vi "Init Waveform.vi"(8 "error in (no error)":errorcluster, 11 "DAQmx Synthesizer in":refnum<class "DAQmx Synthesizer.lvclass">) -> (0 "error out":errorcluster, 3 "DAQmx Synthesizer out":refnum<class "DAQmx Synthesizer.lvclass">)   [LabVIEW 2021, in "DAQmx Synthesizer.lvclass"]
uses:
  DAQmx Synthesizer.lvclass
  DAQmx Synthesizer.lvclass/DAQmx Synthesizer.ctl
  <vilib>/Waveform/WDTOps.llb/WDT Waveform Duration DBL.vi
  <vilib>/Waveform/WDTOps.llb/WDT Get Waveform Subset DBL.vi
panel:
  out "actual duration":dbl format="%0.2f"
  out "actual start samples/time":dbl format="%0.2f"
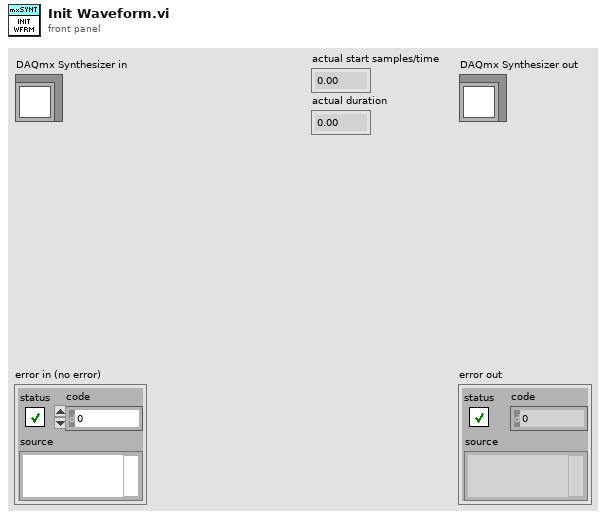
[diagram p1: front panel]
types:
  T1 = enum16{"open", "open or create", "create or replace", "create", "open (read-only)"}
  T2 = typedef "DAQmx Synthesizer Configuration.ctl" = cluster{"Channel names":string[], "Waveform file":path, "Ranges":dbl[], "Post-trigger delay":dbl, "Post-trigger duration":dbl, "Rate":dbl, "Re-name channels":string[], "Active channels":string, "External\nclock":bool, "Group name":string}
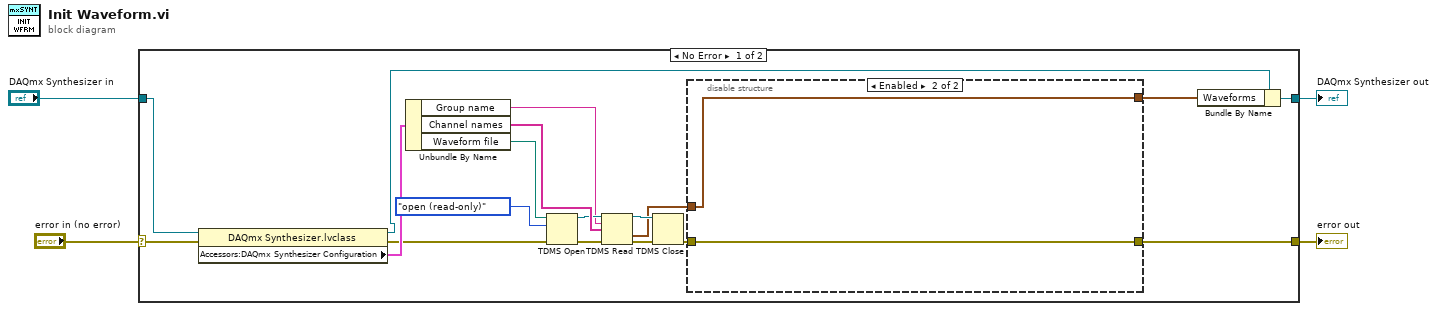
[diagram p0: block diagram]
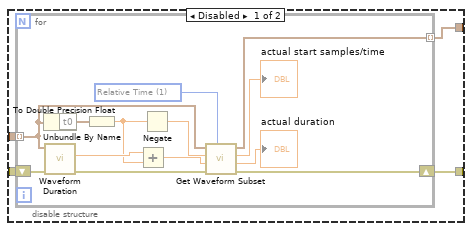
[diagram p2: hidden frame]
diagram:
  n1 = case shown="No Error" "error in (no error)" {
    selector: "error in (no error)" -> [w22 w43]
    tunnel: [w7 w43] -> w3
    tunnel: [w11 w42] -> w1
    tunnel: "DAQmx Synthesizer in" -> [w21 w42]
    frame No Error {
      n2 = property class="DAQmx Synthesizer.lvclass"(reference=w21, error in=w22) -> (reference out=w20:refnum<class "DAQmx Synthesizer.lvclass">, error out=w16:errorcluster, "Accessors:DAQmx Synthesizer Configuration"=w19:T2)
      n3 = Unbundle By Name(w19) -> ("Group name"=w5:string, "Channel names"=w15:string[], "Waveform file"=w18:path)
      n4 = TDMS Open(8:w16, 10:T1."open (read-only)" ("operation (0:open)"), 11:w18) -> (0:w14:errorcluster, 3:w6:refnum<k34>)  [unwired: 4 in]
      n5 = TDMS Read(0:w6, 5:w5, 7:w15, 11:w14) -> (4:w13:refnum<k34>, 10:w9:waveform(dbl)[], 15:w12:errorcluster)  [unwired: 4 in, 3 out]
      n6 = TDMS Close(8:w12, 11:w13) -> (0:w8:errorcluster)  [unwired: 1 out]
      n7 = disable-structure shown="Enabled" {
        disable-tunnel: [w26 w40] -> w10
        disable-tunnel: w9 -> [w25 w40]
        disable-tunnel: w8 -> [w24 w41]
        disable-tunnel: [w23 w41] -> w7
        frame Disabled {
          n8 = for {
            tunnel: w25 -> [w37] mode=indexing
            shift-right: [w39] -> w23
            shift-left: w24 -> [w28]
            tunnel: [w38] -> w26 mode=indexing
            w31 = u16 1 items=["Samples", "Relative Time"] ("start/duration format")
            n9 = Unbundle By Name(w37) -> ("t0"=w34:timestamp)
            n10 = call-poly <vilib>:"Waveform Duration.vi"("error in (no error)"=w28, "waveform in"=w37) -> ("error out"=w27:errorcluster, "duration"=w36:dbl)  [unwired: 7 in, 1 out]
            n11 = To Double Precision Float(number=w34) -> (double precision float=w30:dbl)
            n12 = Add(x=w36, y=w30) -> (x+y=w35:dbl)
            n13 = Negate(x=w30) -> (-x=w29:dbl)
            n14 = call-poly <vilib>:"Get Waveform Subset.vi"("start/duration format"=w31, "error in (no error)"=w27, "duration"=w35, "start samples/time"=w29, "waveform in"=w37) -> ("error out"=w39:errorcluster, "actual duration"=→"actual duration":dbl, "actual start samples/time"=→"actual start samples/time":dbl, "waveform out"=w38:waveform(dbl))  [unwired: 1 in]
          }
        }
        frame Enabled {
        }
      }
      n15 = Bundle By Name(cluster=w20, "Waveforms"=w10) -> (w11:refnum<class "DAQmx Synthesizer.lvclass">)
    }
    frame Error {
    }
  }
  "error out" <- w3
  "DAQmx Synthesizer out" <- w1
